vi "StahlPS_Pbus.CreateServices.vi"(0 "i ref in":refnum<vi>, 5 "error in(no error)":errorcluster) -> (14 "i ref out":refnum<vi>, 19 "error out":errorcluster)   [LabVIEW 2014, in "StahlPS_Pbus.lvlib"]
doc: "This VI Creates two kinds of Services.\n\n1. Monitor services For the GUI, all Values there, are not-Raw Values.\n2. Set - Services for the DSCIntProc, all(most) values there are raw-values."
uses:
  StahlPS_Pbus.lvlib
  CSlibraries-extern/DimLVEvent/LVDimInterface/LVDimInterface.lvlib
  CSCore/CSSystem/CSSystemLib/CSSystemLib.lvlib
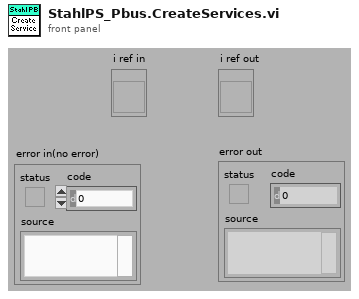
[diagram p1: front panel]
types:
  T1 = typedef "StahlPS_Pbus.lvlib/StahlPS_Pbus.i attribute.ctl" = cluster{"Type":string, "CALC_FACTOR_SET_VOLTAGE":dbl, "CALC_FACTOR_GET_VOLTAGE":dbl, "CALC_FACTOR_GET_CURRENT":dbl, "CALC_FACTOR_SET_CURRENT ":dbl, "REG_VALUE":dbl, "Sign":bool, "setVoltIDs":i32[], "Elektrode Names":string[]}
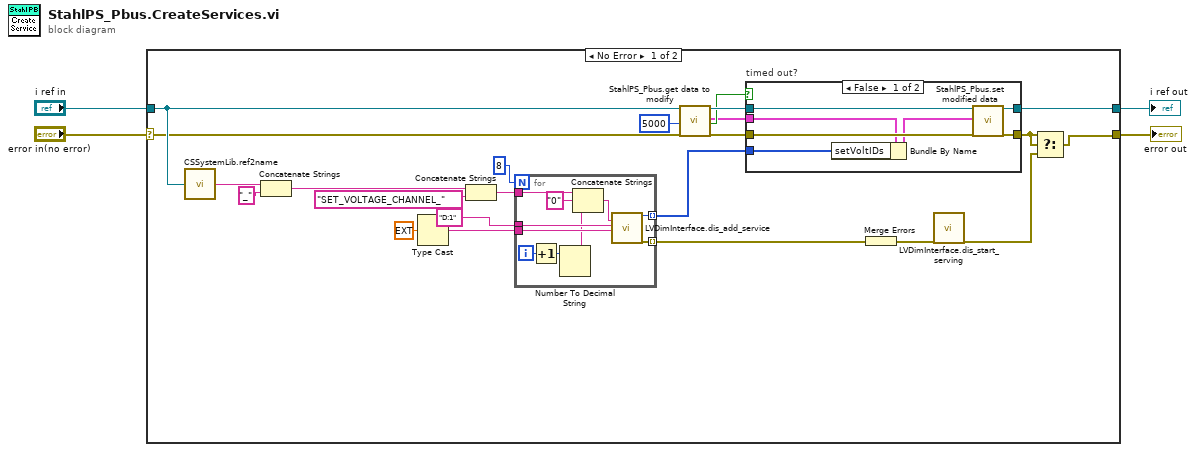
[diagram p0: block diagram]
diagram:
  n1 = case shown="No Error" "error in(no error)" {
    selector: "error in(no error)" -> [w12 w48]
    tunnel: [w16 w48] -> w1
    tunnel: "i ref in" -> [w13 w47]
    tunnel: [w27 w47] -> w2
    frame No Error {
      n2 = call "CSSystemLib.ref2name.vi"("obj refnum"=w13) -> ("name"=w20:string)
      n3 = Concatenate Strings(w20, "_" ("string")) -> (w21:string)
      n4 = Type Cast(x=ext 0.0) -> (*(type *) &x=w24:string)  [unwired: 1 in]
      n5 = Concatenate Strings(w21, "SET_VOLTAGE_CHANNEL_") -> (w7:string)
      n6 = for {
        N: 8 -> [_]
        tunnel: "D:1" ("typeDescriptor") -> [w37]
        tunnel: w24 -> [w36]
        tunnel: [w35] -> w5 mode=indexing
        tunnel: [w34] -> w8 mode=indexing
        tunnel: w7 -> [w33]
        i -> [w31]
        n7 = Increment(x=w31) -> (x+1=w30:i32)
        n8 = Number To Decimal String(number=w30) -> (decimal integer string=w29:string)  [unwired: 1 in]
        n9 = Concatenate Strings(w33, "0" ("string"), w29) -> (w32:string)
        n10 = call "LVDimInterface.dis_add_service.vi"("serviceName"=w32, "typeDescriptor"=w37, "data"=w36) -> ("my_serviceID"=w34:i32, "error out"=w35:errorcluster)  [unwired: 15 in]
      }
      n11 = call "StahlPS_Pbus.get data to modify.vi"("i ref in"=w13, "ms timeout (10000)"=5000, "error in (no error)"=w12) -> ("i ref out"=w19:refnum<vi>, "i attribute"=w11:T1, "timed out"=w14:bool, "error out"=w18:errorcluster)  [unwired: 13 in]
      n12 = case "timed out?" shown="False" w14 {
        tunnel: [w44 w46] -> w27
        tunnel: w19 -> [w43 w46]
        tunnel: w18 -> [w42 w45]
        tunnel: [w41 w45] -> w17
        tunnel: w11 -> [w40 _]
        tunnel: w8 -> [w38 _]
        frame False {
          n13 = Bundle By Name(cluster=w40, "setVoltIDs"=w38) -> (w39:T1)
          n14 = call "StahlPS_Pbus.set modified data.vi"("i ref in"=w43, "i attribute"=w39, "error in (no error)"=w42) -> ("i ref out"=w44:refnum<vi>, "error out"=w41:errorcluster)  [unwired: 15 in]
        }
        frame True {
        }
      }
      n15 = Merge Errors(w5) -> (w10:errorcluster)
      n16 = call "LVDimInterface.dis_start_serving.vi"("error in (no error)"=w10) -> ("error out"=w9:errorcluster)  [unwired: 17 in, 1 out]
      n17 = Select(t=w17, s=w17, f=w9) -> (s? t:f=w16:errorcluster)
    }
    frame Error {
    }
  }
  "error out" <- w1
  "i ref out" <- w2
